vi "Read Challenge Data.vi"(8 "error in (no error)":errorcluster) -> (0 "error out":errorcluster, 2 "Word List":string[](array[string]), 3 "Grid":string[][](array[string]))   [LabVIEW 2024, in "Wordle Scorer.lvlib"]
uses:
  Wordle Scorer.lvlib
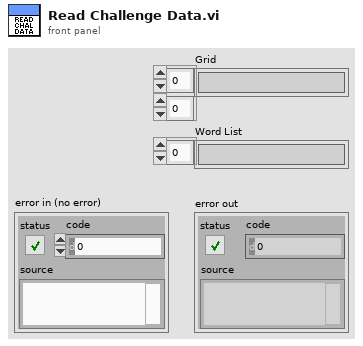
[diagram p1: front panel]
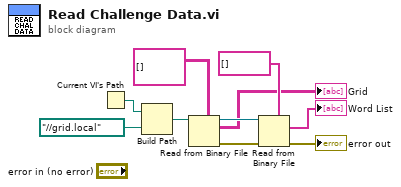
[diagram p0: block diagram]
diagram:
  n1 = Current VI's Path() -> (path=w10:path)
  n2 = Build Path(base path=w10, name or relative path=path "../../grid.local") -> (appended path=w8:path)
  n3 = Read from Binary File(5:string[][] [] ("Grid"), 11:w8) -> (0:w5:errorcluster, 2:→"Grid":string[][], 3:w4:refnum<file>)  [unwired: 4 in, 1 out]
  n4 = Read from Binary File(5:string[] [], 8:w5, 11:w4) -> (0:→"error out":errorcluster, 2:→"Word List":string[])  [unwired: 3 in, 2 out]
